vi "HOST_8wave.vi"() -> ()   [LabVIEW 2020]
uses:
  <vilib>/userDefined/Silver/nirio_resource_slv.ctl
  Controls/Clock Select.ctl
  <vilib>/FPGAPlugInAG/PXIe-7972R/niLvFpga_Open_PXIe-7972R.vi
  <vilib>/rvi/interface/common/dynamic/niFpgaDynamicAddResources.vi
  <vilib>/rvi/interface/common/niFpgaWaitOnOcc.vi
  <vilib>/Utility/error.llb/Error Cluster From Error Code.vi
  <vilib>/rvi/errors/niLvFpgaAdjustHostInterfaceError.vi
  <instrlib>/_niInstr/Streaming/v1/Host/Public/Start Finite Stream.vi
  <instrlib>/_niInstr/Streaming/v1/Host/Public/Wait for Stream.vi
  <instrlib>/_niInstr/Streaming/v1/Host/Public/Start Continuous Stream.vi
  <vilib>/FPGAPlugInAG/Dynamic/niLvFpga_Close_Dynamic.vi
  <vilib>/rvi/interface/nirviOpenFPGA/nirviOpenFPGA.xnode
  FPGA Bitfiles/rfsignal_FPGATarget_8waves_NONOGDFcqUo.lvbitx
  <vilib>/rvi/interface/nirviMethod/nirviMethod.xnode
  <vilib>/rvi/interface/nirviReadWriteControl/nirviReadWriteControl.xnode
  <vilib>/rvi/interface/nirviCloseFPGA/nirviCloseFPGA.xnode
  <vilib>/rvi/errors/niLvFpgaMergeErrorWithErrorCode.vi
  <instrlib>/_niInstr/Streaming/v1/Host/niInstr Streaming v1 Host.lvlib
  <vilib>/rvi/interface/Simulation/niFpgaSimulationCallBeginRW.vi
  <vilib>/FPGAPlugInAG/Dynamic/niLvFpga_ConfigureFifo_Dynamic.vi
  <vilib>/FPGAPlugInAG/Dynamic/niLvFpga_StartFifo_Dynamic.vi
  NiFpgaLv.dll
  <vilib>/FPGAPlugInAG/Dynamic/niLvFpga_WriteFifo_Dynamic.vi
panel:
  out "AO":waveform(dbl)(graph)={"t0"=timestamp(0.013800004999999999 s since 1904-01-01), "dt"=1e-08, "Y"=array[60000 elements]}
  in  "Wave reader":fxp<+,32,10>[](array[numeric])
  in  "?":bool
  out "Numeric":i32=7
  in  "Wave On":bool[](array[boolean])=[TRUE, FALSE, FALSE, FALSE, FALSE, FALSE, FALSE, FALSE]
  in  "Amplitude (V)":dbl[](array[numeric])=[0.1, 0.12, 0.12, 0.12, 0.1, 0.12, 0.12, 0.12] format="%0.2p"
  in  "Frequencies (Hz)":dbl[](array[numeric])=[27000000.0, 2000000.0, 3000000.0, 4000000.0, 27000000.0, 6000000.0, 7000000.0, 8000000.0] format="%5p"
  in  "Rate":fxp<+,32,10>
  in  "Loop time (ms)":u32=5
  in  "Signal Type":T1(ring)
  in  "Dynamic 2":fxp<+,32,10>
  in  "Dynamic 1":fxp<+,32,10>
  in  "Sampling Info":cluster{"Fs":dbl, "#s":dbl}={"Fs"=100000000.0, "#s"=60000.0} {"Fs" format="%#_3p"}
  out "Error Out":errorcluster
  in  "Update Waveform":bool
  in  "AO Channel":T2(ring)
  in  "Clock Select":T3 items=["Internal Clock", "Internal Clock w/ Ref via CLK/REF IN", "Internal Clock w/ Ref via Sync Clock", "External Clock via CLK/REF IN"]
  in  "Rate of External Sample Clock (MHz)":u16=100 min=60 max=100 step=1
  in  "RIO Resource":T4="RIO0"
  # "CH1"
  # "Don't change"
  # "CH2"
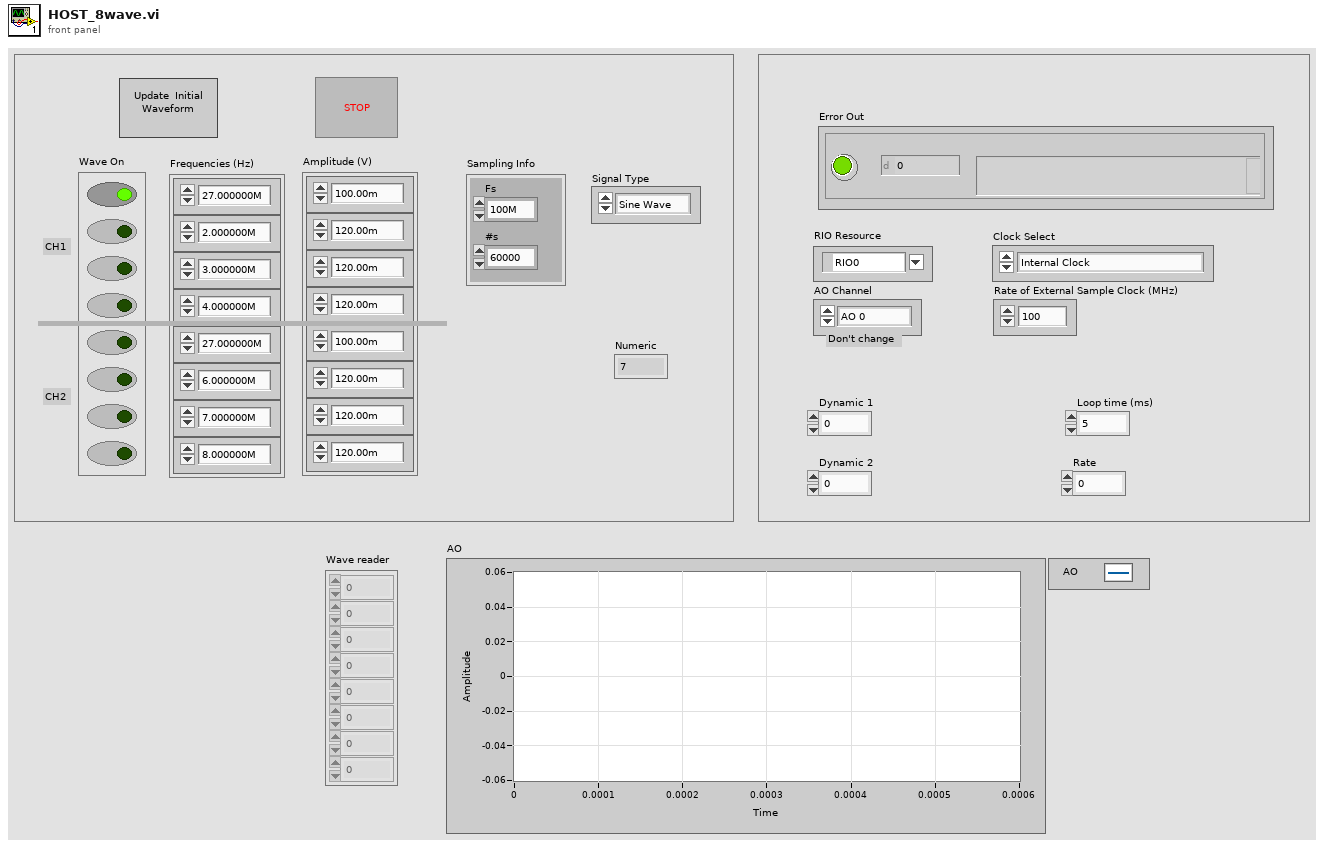
[diagram p1: front panel]
types:
  T1 = enum16{"Sine Wave", "Triangle Wave", "Square Wave", "Sawtooth Wave"}
  T2 = enum8{"AO 0", "AO 1", "AO 2", "AO 3", "AO 0, AO 1, AO 2, AO 3", "None"}
  T3 = typedef "Clock Select.ctl" = u16
  T4 = typedef "nirio_resource_slv.ctl" = tag
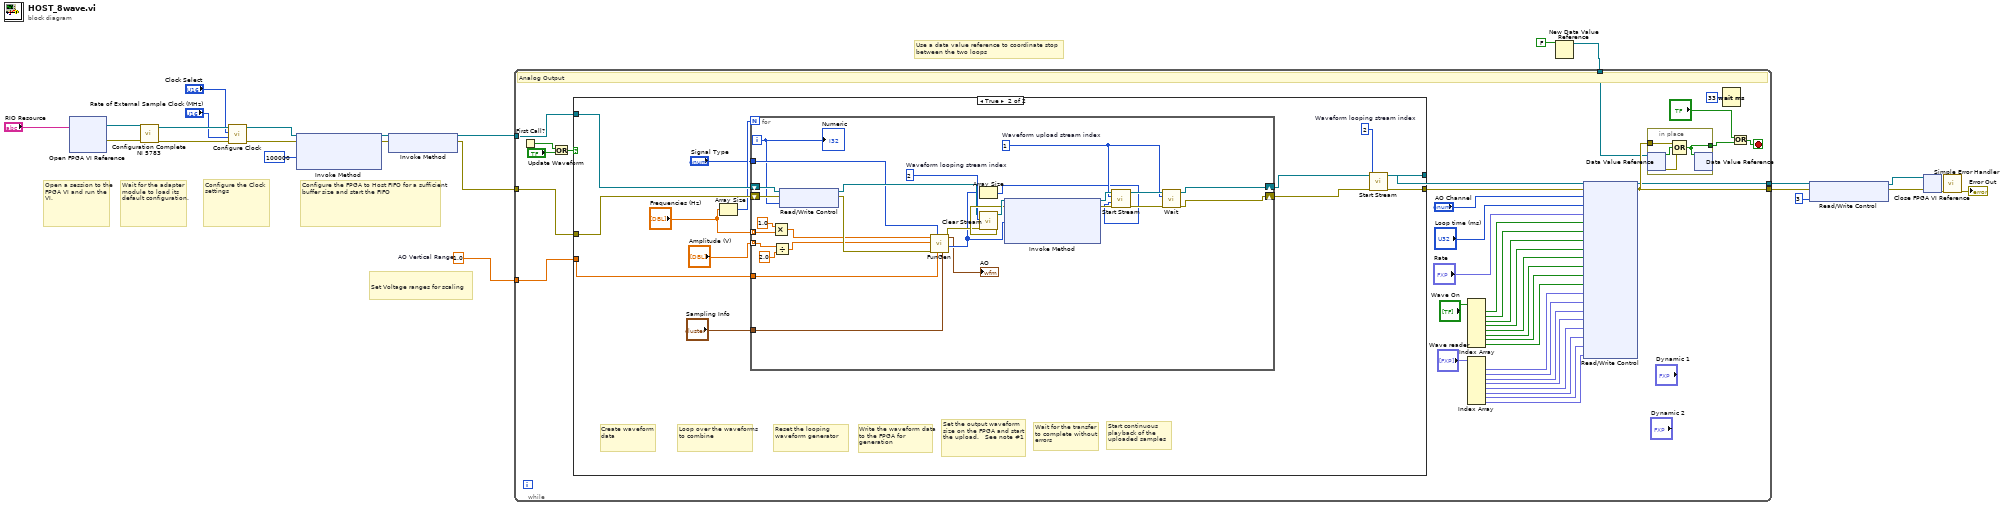
[diagram p0: block diagram]
diagram:
  w9 = 1.0  # AO Vertical Range
  # "Use a data value reference to coordinate stop between the two loops"
  # "Set Voltage ranges for scaling"
  # "Configure the Clock settings"
  # "Configure the FPGA to Host FIFO for a sufficient buffer size and start the FIFO"
  # "Wait for the adapter module to load its default configuration."
  # "Open a session to the FPGA VI and run the VI."
  n1 = xnode "Open FPGA VI Reference"("resource name"="RIO Resource") -> ("FPGA VI Reference Out"=w7:refnum<k20>, "error out"=w6:errorcluster)  [unwired: 1 in]
  n2 = call "Configuration Complete NI 5783.vi"("error in"=w6, "FPGA VI Reference In"=w7) -> ("error out"=w20:errorcluster, "FPGA VI Reference Out"=w21:refnum<k20>)  [unwired: 7 in, 1 out]
  n3 = call "Configure Clock.vi"("error in (no error)"=w20, "Rate of External Sample Clock (MHz)"="Rate of External Sample Clock (MHz)", "Clock Select"="Clock Select", "FPGA VI Reference In"=w21) -> ("error out"=w18:errorcluster, "FPGA VI Reference Out"=w19:refnum<k20>)  [unwired: 3 in, 3 out]
  n4 = xnode "Invoke Method"("FPGA VI Reference In"=w19, "error in"=w18, "Requested Depth"=u32 100000) -> ("FPGA VI Reference Out"=w24:refnum<k20>, "error out"=w23:errorcluster)  [unwired: 1 out]
  n5 = xnode "Invoke Method"("FPGA VI Reference In"=w24, "error in"=w23) -> ("FPGA VI Reference Out"=w15:refnum<k20>, "error out"=w14:errorcluster)
  n6 = New Data Value Reference(data value=FALSE ("Stopped")) -> (data value reference=w10:refnum<data-value>)  [unwired: 1 in, 1 out]
  n7 = while {
    tunnel: w14 -> [w52]
    tunnel: [w57] -> w5
    tunnel: w15 -> [w60]
    tunnel: [w54] -> w4
    tunnel: w10 -> [w53]
    tunnel: w9 -> [w51]
    stop <- w37 stop-if-true
    # "Analog Output"
    n8 = First Call?() -> (First Call?: T/F=w55:bool)
    n9 = Or(x=w55, y="Update Waveform") -> (x .or. y?=w56:bool)
    n10 = case shown="True" w56 {
      tunnel: [w66 w79] -> w50
      tunnel: [w65 w78] -> w49
      tunnel: w60 -> [w66 w76]
      tunnel: w52 -> [w65 w75]
      tunnel: w51 -> [_ w77]
      frame False {
      }
      frame True {
        w74 = 2  # Waveform looping stream index
        # "Loop over the waveforms to combine"
        # "Reset the looping waveform generator"
        # "Start continuous playback of the uploaded samples"
        # "Wait for the transfer to complete without errors"
        # "Set the output waveform size on the FPGA and start the upload.   See note #1"
        # "Write the waveform data to the FPGA for generation"
        # "Create waveform data"
        n11 = Array Size(array="Frequencies (Hz)") -> (size(s)=w69:i32)
        n12 = for {
          N: w69 -> [_]
          tunnel: w77 -> [w97]
          shift-right: [w89] -> w73
          shift-left: w76 -> [w96]
          shift-right: [w88] -> w72
          shift-left: w75 -> [w94]
          tunnel: "Frequencies (Hz)" -> [w87] mode=indexing
          tunnel: "Amplitude (V)" -> [w83] mode=indexing
          tunnel: "Sampling Info" -> [w86]
          tunnel: "Signal Type" -> [w85]
          i -> [w84]
          w98 = 2  # Waveform looping stream index
          w103 = 1  # Waveform upload stream index
          n13 = Multiply(x=1.0, y=w87) -> (x*y=w91:dbl)
          n14 = Divide(x=w83, y=2.0) -> (x/y=w82:dbl)
          n15 = xnode "Read/Write Control"("FPGA VI Reference In"=w96, "error in"=w94, "Upload selector"=w84) -> ("FPGA VI Reference Out"=w95:refnum<k20>, "error out"=w93:errorcluster)
          n16 = call "FunGen.vi"("sampling info"=w86, "range (Vpp)"=w97, "signal type"=w85, "error in (no error)"=w93, "amplitude"=w82, "frequency"=w91) -> ("error out"=w99:errorcluster, "Waveform Data"=w90:i16[], "Output Waveform (V)"=→"AO":waveform(dbl))  [unwired: 2 in, 1 out]
          n17 = Array Size(array=w90) -> (size(s)=w100:i32)
          n18 = call <instrlib>:"Clear Stream.vi"("error in (no error)"=w99, "stream index"=w98, "refnum in"=w95) -> ("error out"=w101:errorcluster, "refnum out"=w102:refnum<k20>)  [unwired: 7 in]
          n19 = xnode "Invoke Method"("FPGA VI Reference In"=w102, "error in"=w101, "Data"=w90) -> ("FPGA VI Reference Out"=w107:refnum<k20>, "error out"=w106:errorcluster)  [unwired: 1 in, 1 out]
          n20 = call-poly <instrlib>:"Start Stream.vi"("error in (no error)"=w106, "num samples"=w100, "stream index"=w103, "refnum in"=w107) -> ("error out"=w104:errorcluster, "refnum out"=w105:refnum<k20>)  [unwired: 6 in]
          n21 = call-poly <instrlib>:"Wait.vi"("error in (no error)"=w104, "stream index"=w103, "refnum in"=w105) -> ("error out"=w88:errorcluster, "refnum out"=w89:refnum<k20>)  [unwired: 5 in, 2 out]
          "Numeric" <- w84
        }
        n22 = call-poly <instrlib>:"Start Stream.vi"("error in (no error)"=w72, "stream index"=w74, "refnum in"=w73) -> ("error out"=w78:errorcluster, "refnum out"=w79:refnum<k20>)  [unwired: 7 in]
      }
    }
    n23 = Index Array(array="Wave reader") -> (element #1=w32:fxp<+,32,10>, element #2=w31:fxp<+,32,10>, element #3=w30:fxp<+,32,10>, element #4=w29:fxp<+,32,10>, element #5=w28:fxp<+,32,10>, element #6=w27:fxp<+,32,10>, element #7=w26:fxp<+,32,10>, element #8=w25:fxp<+,32,10>)  [unwired: 8 in]
    n24 = Index Array(array="Wave On") -> (element #1=w44:bool, element #2=w38:bool, element #3=w39:bool, element #4=w40:bool, element #5=w41:bool, element #6=w42:bool, element #7=w43:bool, element #8=w33:bool)  [unwired: 8 in]
    n25 = xnode "Read/Write Control"("FPGA VI Reference In"=w50, "error in"=w49, "AO Channel"="AO Channel", "Time (milisec)"="Loop time (ms)", "Rate"="Rate", "Wave On 1"=w44, "Wave On 2"=w38, "Wave On 3"=w39, "Wave On 4"=w40, "Wave On 5"=w41, "Wave On 6"=w42, "Wave On 7"=w43, "Wave On 8"=w33, "Wave 1"=w32, "Wave 2"=w31, "Wave 3"=w30, "Wave 4"=w29, "Wave 5"=w28, "Wave 6"=w27, "Wave 7"=w26, "Wave 8"=w25) -> ("FPGA VI Reference Out"=w54:refnum<k20>, "error out"=w57:errorcluster)
    n26 = in-place {
      in-place-border: [w62] -> w36
      in-place-border: w57 -> [w64]
      n27 = in-place-dvr #1(w53) -> (w63:bool, w61:errorcluster)
      n28 = Compound Arithmetic op=OR(w64, w63, w61) -> (w62:bool)
      n29 = in-place-dvr #1(w62) -> ()  [unwired: 2 out]
    }
    n30 = Wait (ms)(milliseconds to wait=u32 33) -> ()  [unwired: 1 out]
    n31 = Or(x="?", y=w36) -> (x .or. y?=w37:bool)
  }
  n32 = xnode "Read/Write Control"("FPGA VI Reference In"=w4, "error in"=w5, "stream.request state 2"=3) -> ("FPGA VI Reference Out"=w1:refnum<k20>, "error out"=w3:errorcluster)
  n33 = xnode "Close FPGA VI Reference"("FPGA VI Reference In"=w1, "error in"=w3) -> ("error out"=w13:errorcluster)
  n34 = call <vilib>:"Simple Error Handler.vi"("error in (no error)"=w13) -> ("error out"=→"Error Out":errorcluster)  [unwired: 4 in, 4 out]
